vi "Error Query.vi"(0 "VISA resource name":refnum<visa-resource-name>, 11 "error in (no error)":errorcluster) -> (4 "VISA resource name out":refnum<visa-resource-name>, 8 "Error Code":i32, 10 "Error Message":string, 15 "error out":errorcluster)   [LabVIEW 2014, in "Fluke 5XXX Series Multicalibrators.lvlib"]
doc: "This VI reads an error from the instrument. It expects to see errors in SCPI format (#,\"error message\"). If an error query is not supported, it returns a warning."
uses:
  Fluke 5XXX Series Multicalibrators.lvlib
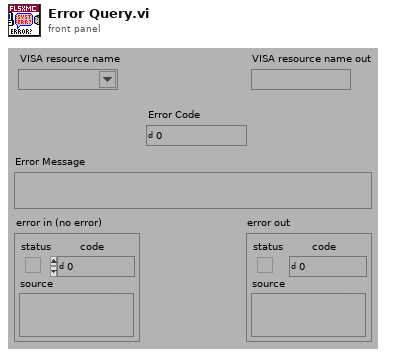
[diagram p1: front panel]
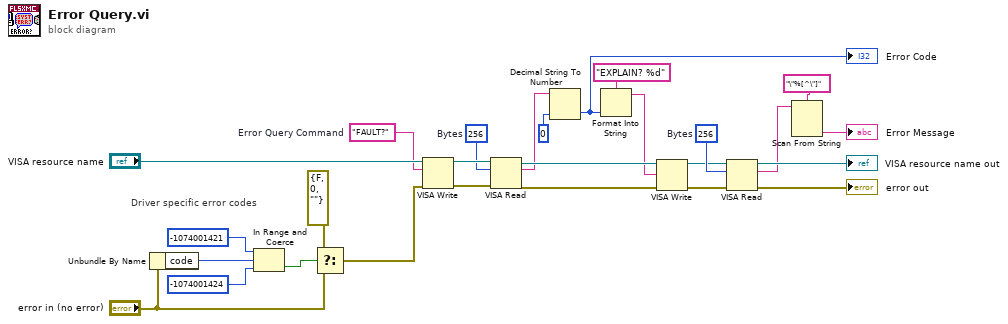
[diagram p0: block diagram]
diagram:
  w21 = u32 256  # Bytes
  w25 = u32 256  # Bytes
  w23 = "FAULT?"  # Error Query Command
  # "Driver specific error codes"
  n1 = Unbundle By Name("error in (no error)") -> ("code"=w6:i32)
  n2 = In Range and Coerce(upper limit=-1074001421, x=w6, lower limit=-1074001424) -> (In Range?=w5:bool)  [unwired: 1 out]
  n3 = Select(t=errorcluster {"status"=FALSE, "code"=0, "source"=""} ("error out"), s=w5, f="error in (no error)") -> (s? t:f=w2:errorcluster)
  n4 = VISA Write(VISA resource name="VISA resource name", write buffer=w23, error in (no error)=w2) -> (VISA resource name out=w26:refnum<visa-resource-name>, error out=w24:errorcluster)  [unwired: 1 out]
  n5 = VISA Read(VISA resource name=w26, byte count=w25, error in (no error)=w24) -> (VISA resource name out=w16:refnum<visa-resource-name>, read buffer=w13:string, error out=w19:errorcluster)  [unwired: 1 out]
  n6 = Decimal String To Number(string=w13, default (0L)=0) -> (number=w12:i32)  [unwired: 1 in, 1 out]
  "Error Code" <- w12
  n7 = Format Into String(format string="EXPLAIN? %d", w12) -> (resulting string=w15:string)  [unwired: 2 in, 1 out]
  n8 = VISA Write(VISA resource name=w16, write buffer=w15, error in (no error)=w19) -> (VISA resource name out=w20:refnum<visa-resource-name>, error out=w22:errorcluster)  [unwired: 1 out]
  n9 = VISA Read(VISA resource name=w20, byte count=w21, error in (no error)=w22) -> (VISA resource name out=→"VISA resource name out":refnum<visa-resource-name>, read buffer=w10:string, error out=→"error out":errorcluster)  [unwired: 1 out]
  n10 = Scan From String(format string="\"%[^\"]" ("Format String"), input string=w10) -> (output 1=→"Error Message":string)  [unwired: 3 in, 3 out]
